vi "PCO_GetCmosLineTiming.vi"(0 "ph":u64, 5 "error in (no error)":errorcluster {"code" format="%x"}) -> (10 "minLineTime_ns":u32, 11 "maxLineTime_ms":u32, 14 "ph out":u64, 15 "ErrorMessage":i32 format="%x", 16 "wParameter":u16(ring) items=["OFF", "ON"], 17 "dwLineTime":u32, 18 "wTimeBase":u16(ring) items=["ns", "us", "ms"], 19 "error out":errorcluster {"code" format="%x"})   [LabVIEW 2019, in "SDK.lvlib" / "SpecialCommandsEdge.lvlib"]
doc: "<b>Description:</b>\nThis function returns the current settings of the Lightsheet scanning mode of the pco.edge.\nIf this mode is active, timing related settings from the functions in TIMING CONTROL are inactive and current delay and exposure times must be readout with function PCO_GetCmosLineExposureDelay.\nThe resulting exposure time in £gs can be calculated as:\nint64 expos=dwExposureLines*dwLineTime*(1000.dwTimebase).\n\n<b>Supported camera type:</b>\npco.edge with Camera Link interface\n\n<b>Descriptor dependency:</b>\nNone"
uses:
  SpecialCommandsEdge.lvlib
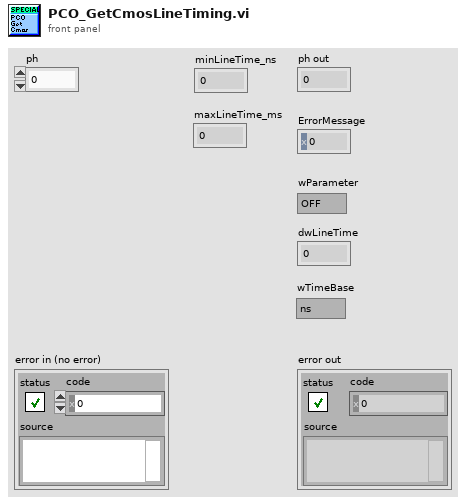
[diagram p1: front panel]
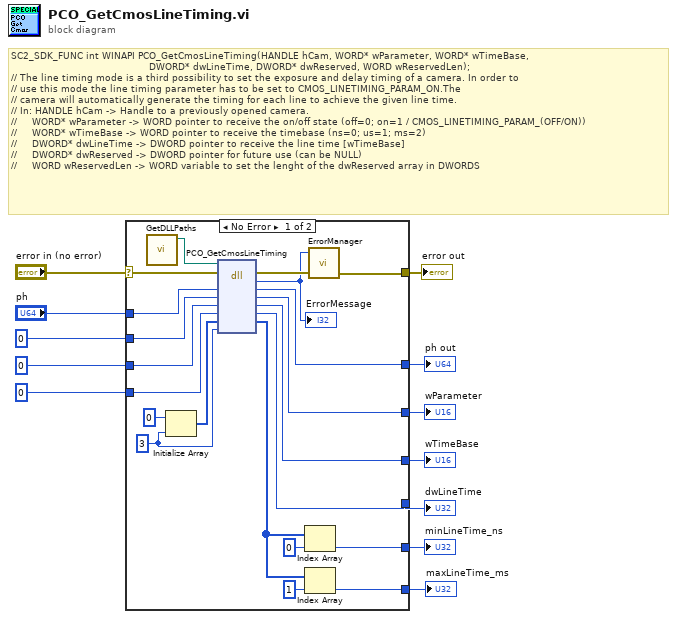
[diagram p0: block diagram]
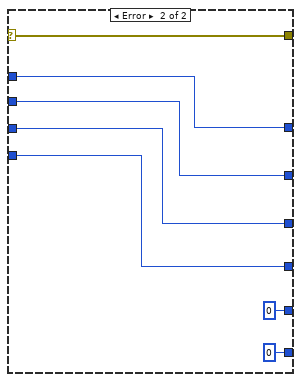
[diagram p2: hidden frame]
diagram:
  # "SC2_SDK_FUNC int WINAPI PCO_GetCmosLineTiming(HANDLE hCam, WORD* wParameter, WORD* wTimeBase,\n                                              DWORD* dwLineTime, DWORD* dwReserved, WORD wReservedLen);\n// The line timing mode is a third possibility to set the exposure and delay timing of a camera. In order to \n// use this mode the line timing parameter has to be set to CMOS_LINETIMING_PARAM_ON.The\n// camera will automatically generate the timing for each line to achieve the given line time.\n// In: HANDLE hCam -> Handle to a previously opened camera.\n//     WORD* wParameter -> WORD pointer to receive the on/off state (off=0; on=1 / CMOS_LINETIMING_PARAM_(OFF/ON))\n//     WORD* wTimeBase -> WORD pointer to receive the timebase (ns=0; us=1; ms=2)\n//     DWORD* dwLineTime -> DWORD pointer to receive the line time [wTimeBase]\n//     DWORD* dwReserved -> DWORD pointer for future use (can be NULL)\n//     WORD wReservedLen -> WORD variable to set the lenght of the dwReserved array in DWORDS"
  n1 = case shown="No Error" "error in (no error)" {
    selector: "error in (no error)" -> [w22 w40]
    tunnel: "ph" -> [w33 w39]
    tunnel: [w32 w39] -> w11
    tunnel: [w31 w38] -> w10
    tunnel: [w30 w37] -> w9
    tunnel: u32 0 ("dwLineTime") -> [w29 w36]
    tunnel: [w28 w36] -> w7
    tunnel: [w20 w40] -> w6
    tunnel: u16 0 ("wParameter") -> [w24 w38]
    tunnel: u16 0 ("wTimeBase") -> [w23 w37]
    tunnel: [w14 u32 0] -> w2
    tunnel: [w13 u32 0] -> w1
    frame No Error {
      w25 = u16 3 ("dimension size")
      n2 = call "GetDLLPaths.vi"() -> ("SC2_Cam_Path"=w18:path)  [unwired: 8 in, 3 out]
      n3 = Initialize Array(u32 0, w25) -> (w26:u32[])
      n4 = dll-call lib="?" fn="PCO_GetCmosLineTiming"(path in=w18, error in=w22, "ph"=w33, "wParameter"=w24, "wTimeBase"=w23, "dwLineTime"=w29, "dwReserved"=w26, "wReservedLen"=w25) -> (error out=w21:errorcluster, "return type"=w19:i32, "ph"=w32:u64, "wParameter"=w31:u16, "wTimeBase"=w30:u16, "dwLineTime"=w28:u32, "dwReserved"=w15:u32[])  [unwired: 2 in, 1 out]
      "ErrorMessage" <- w19
      n5 = Index Array(array=w15, index=0) -> (element=w14:u32)
      n6 = Index Array(array=w15, index=1) -> (element=w13:u32)
      n7 = call "ErrorManager.vi"("error in (no error)"=w21, "error code"=w19) -> ("error out"=w20:errorcluster)  [unwired: 2 in, 1 out]
    }
    frame Error {
    }
  }
  "ph out" <- w11
  "wParameter" <- w10
  "wTimeBase" <- w9
  "dwLineTime" <- w7
  "error out" <- w6
  "minLineTime_ns" <- w2
  "maxLineTime_ms" <- w1
